vi "Lvi Close Task.vi"(8 "error in (no error)":errorcluster, 11 "TaskRef":i32) -> (0 "error out":errorcluster, 3 "function return":u32(ring))   [LabVIEW 2022 SP3, in "DtLvLink.lvlib"]
doc: "Calls directly into the entry points of the DLL of the Data Acq SDK to stop the task if it is running and release all resources that are associated with the task. This VI is used by the higher-level VI, DtOLCloseTask."
uses:
  DtLvLink.lvlib
  <userlib>/LV-Link3/DtLvLink_64.dll
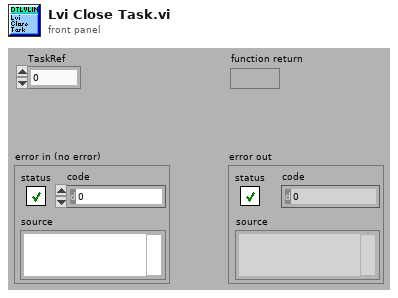
[diagram p1: front panel]
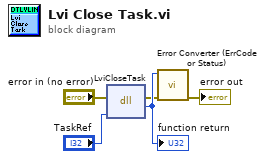
[diagram p0: block diagram]
diagram:
  n1 = dll-call lib="C:/Program Files/National Instruments/LabVIEW 2022/user.lib/LV-Link3/DtLvLink_64.*" fn="LviCloseTask"(error in="error in (no error)", "TaskRef"="TaskRef") -> (error out=w2:errorcluster, w5:u32)  [unwired: 3 in, 1 out]
  "function return" <- w5
  n2 = call "Error Converter (ErrCode or Status).vi"("error in (no error)"=w2, "error code"=w5) -> ("error out"=→"error out":errorcluster)  [unwired: 9 in]
